vi "Build Movement Proposals.vi"() -> (0 "Movement Proposal Rules":T2(array[cluster]))   [LabVIEW 2020, in "AoC 2022.lvlib"]
uses:
  AoC 2022.lvlib
  Day 15 - Beacon Exclusion Zone/private/Location.ctl
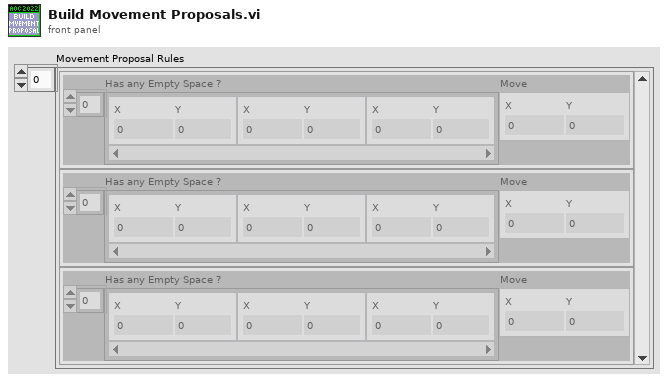
[diagram p1: front panel]
types:
  T1 = typedef "AoC 2022.lvlib/Location.ctl" = cluster{"X":i32, "Y":i32}
  T2 = cluster{"Has any Empty Space ?":T1[], "Move":T1}[]
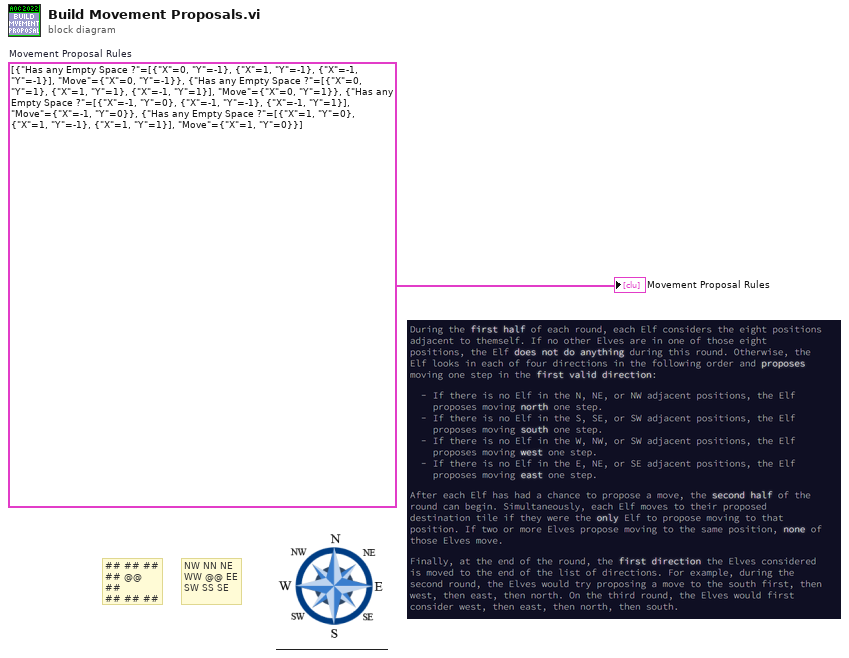
[diagram p0: block diagram]
diagram:
  w1 = T2 [{"Has any Empty Space ?"=[{"X"=0, "Y"=-1}, {"X"=1, "Y"=-1}, {"X"=-1, "Y"=-1}], "Move"={"X"=0, "Y"=-1}}, {"Has any Empty Space ?"=[{"X"=0, "Y"=1}, {"X"=1, "Y"=1}, {"X"=-1, "Y"=1}], "Move"={"X"=0, "Y"=1}}, {"Has any Empty Space ?"=[{"X"=-1, "Y"=0}, {"X"=-1, "Y"=-1}, {"X"=-1, "Y"=1}], "Move"={"X"=-1, "Y"=0}}, {"Has any Empty Space ?"=[{"X"=1, "Y"=0}, {"X"=1, "Y"=-1}, {"X"=1, "Y"=1}], "Move"={"X"=1, "Y"=0}}]  # Movement Proposal Rules
  # "NW NN NE\nWW @@ EE\nSW SS SE"
  # "## ## ##\n## @@ ##\n## ## ##"
  "Movement Proposal Rules" <- w1
